vi "SP Handle Data Display Change.vi"(4 "Cache and New Are Same?":bool, 6 "Queue Cluster":T1={"Command"="", "Test Parameters"={"Stimulus"={"Use Instrument Settings"=FALSE, "Blank Frequencies"=FALSE, "Sweep Type"=enum."Linear", "Sweep"={"Fstart"=500.0, "Fstop"=1500.0, "Units"=enum."MHz", "Points"=2}, "Power (dBm)"=999.0, "IFBW (Hz)"=-1.0, "Sweep Time (s)"=-1.0, "Calibration"={"State"=FALSE, "String"=""}}, "Measurement"={"Auto Select"=TRUE, "Data Source"=enum."VNA", "Ports"=2, "Parameters"=[]}, "De-Embed"={"De-Embed"=FALSE, "Adapters"=[]}, "Display"={"Lock Control"=FALSE, "Retain Settings"=TRUE, "Formatted Data"=FALSE, "Plot Orientation"=enum."Single", "Plot Controls"=[{"Trace Orientation"=enum."Overlay", "Frequency"={"Change Frequency"=FALSE, "Start"=500.0, "Stop"=1500.0, "Units"=enum."MHz"}, "Markers"=[], "Traces"=[]}, {"Trace Orientation"=enum."Overlay", "Frequency"={"Change Frequency"=FALSE, "Start"=500.0, "Stop"=1500.0, "Units"=enum."MHz"}, "Markers"=[], "Traces"=[]}, {"Trace Orientation"=enum."Overlay", "Frequency"={"Change Frequency"=FALSE, "Start"=500.0, "Stop"=1500.0, "Units"=enum."MHz"}, "Markers"=[], "Traces"=[]}, {"Trace Orientation"=enum."Overlay", "Frequency"={"Change Frequency"=FALSE, "Start"=500.0, "Stop"=1500.0, "Units"=enum."MHz"}, "Markers"=[], "Traces"=[]}]}, "Limits"=[], "Filter Limits"=[]}} {"Test Parameters"."Filter Limits"."Parameter"."Stimulus Port" min=1 step=1; "Test Parameters"."Filter Limits"."Parameter"."Response Port" min=1 step=1; "Test Parameters"."Filter Limits"."Passband"."Bandwidth Attn" format="%.3g"; "Test Parameters"."Filter Limits"."Passband"."Stop/Span" format="%.3g"; "Test Parameters"."Filter Limits"."Passband"."Start/Center" format="%.3g"; "Test Parameters"."Measurement"."Parameters"."Channel" min=0 max=32 step=1; "Test Parameters"."Measurement"."Parameters"."Parameter"."Stimulus Port" min=1 step=1; "Test Parameters"."Measurement"."Parameters"."Parameter"."Response Port" min=1 step=1; "Test Parameters"."Limits"."Parameter"."Stimulus Port" min=1 step=1; "Test Parameters"."Limits"."Parameter"."Response Port" min=1 step=1; "Test Parameters"."Stimulus"."Sweep Time (s)" format="%.3g"; "Test Parameters"."Display"."Plot Controls"."Traces"."Reference" format="%#.2g"; "Test Parameters"."Display"."Plot Controls"."Traces"."Scale" min=0.001 step=1.0 format="%#.2g"; "Test Parameters"."Display"."Plot Controls"."Traces"."Position" min=0.0 max=10.0; "Test Parameters"."Display"."Plot Controls"."Frequency"."Stop" format="%.3g"; "Test Parameters"."Display"."Plot Controls"."Frequency"."Start" format="%.3g"}, 8 "error in (no error)":errorcluster, 9 "CH Other":refnum<vi>, 10 "CH Changing":refnum<vi>, 11 "Queue":refnum<queue>) -> (0 "error out":errorcluster, 2 "Plot?":bool)   [LabVIEW 2011]
uses:
  TypeDefs/SP Queue Cluster.ctl
  TypeDefs/SP Test Parameters.ctl
  TypeDefs/SP Stimulus Parameters.ctl
  TypeDefs/SP Frequency Units.ctl
  TypeDefs/SP Calibration State.ctl
  TypeDefs/SP Measurement.ctl
  TypeDefs/SP Parameters.ctl
  TypeDefs/SP Parameter.ctl
  TypeDefs/SP De-Embed.ctl
  TypeDefs/SP Adapter.ctl
  TypeDefs/SP Data.ctl
  TypeDefs/SP Display Parameters.ctl
  TypeDefs/SP Display Plot Controls Cluster.ctl
  TypeDefs/SP Marker Cluster.ctl
  TypeDefs/SP Marker Type.ctl
  TypeDefs/SP Display Trace Controls.ctl
  TypeDefs/SP Display Format.ctl
  TypeDefs/SP Display Data.ctl
  TypeDefs/SP Limit.ctl
  TypeDefs/SP Format.ctl
  TypeDefs/SP Limit Type.ctl
  TypeDefs/SP Limit Point.ctl
  Test Referential Limit.ctl
  TypeDefs/SP Filter.ctl
  TypeDefs/SP Filter Type.ctl
  TypeDefs/SP Filter Passband.ctl
  TypeDefs/SP Frequency Format.ctl
  TypeDefs/SP Filter Ripple.ctl
  TypeDefs/SP Attenuation Point.ctl
  TypeDefs/SP Attenuation Type.ctl
  TypeDefs/SP Skirt Rejection Point.ctl
  TypeDefs/SP Relative Loss.ctl
panel:
  # "Div"
  # "Div"
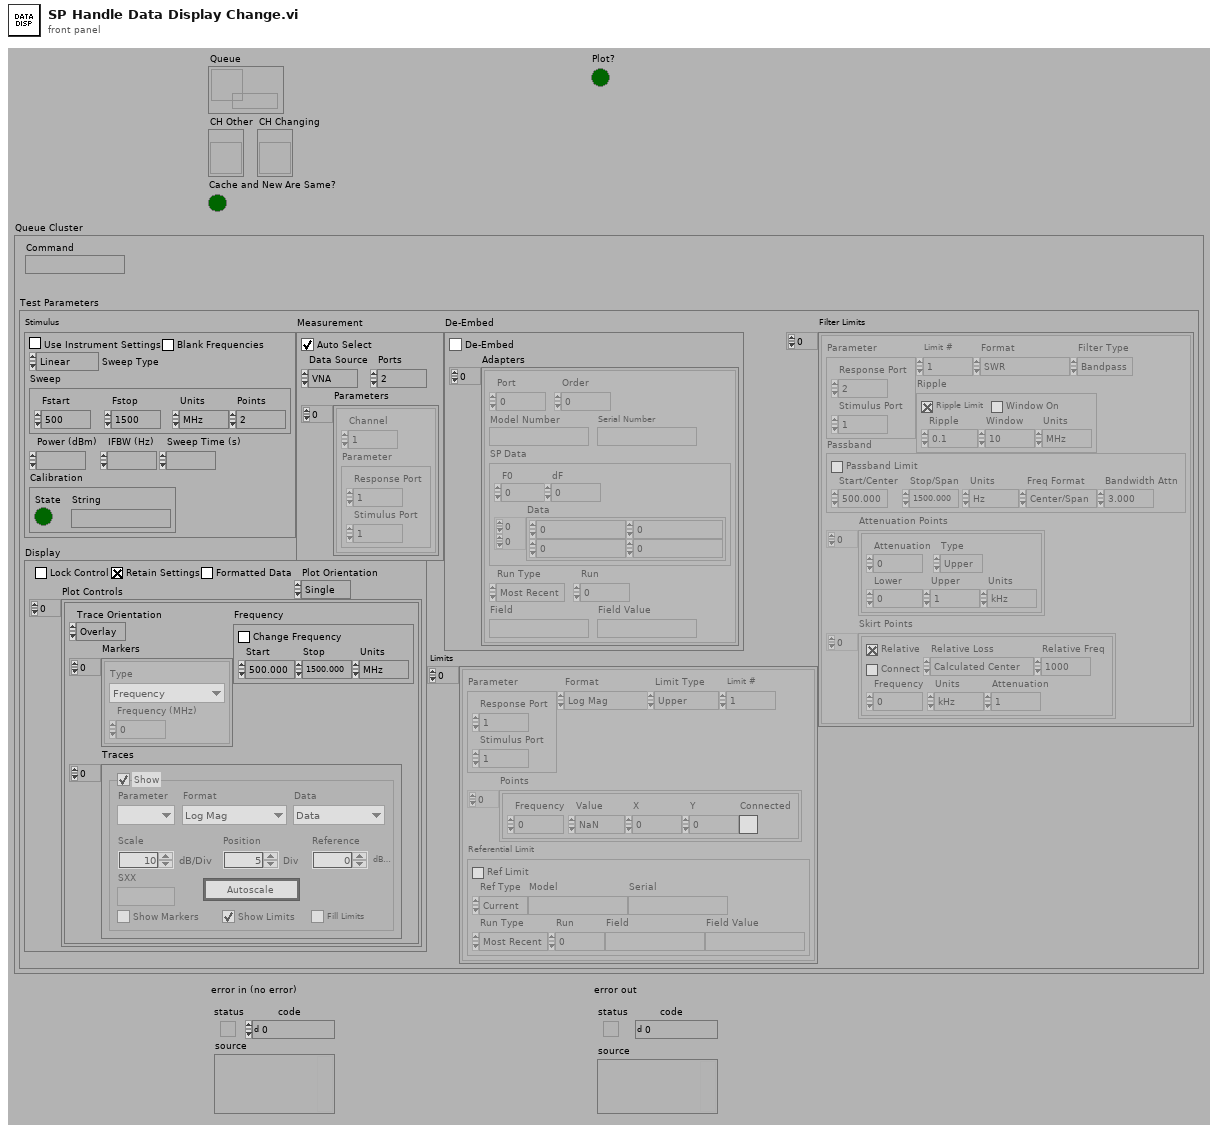
[diagram p1: front panel]
types:
  T1 = typedef "SP Queue Cluster.ctl" = cluster{"Command":string, "Test Parameters":T2}
  T2 = typedef "SP Test Parameters.ctl" = cluster{"Stimulus":T3, "Measurement":T6, "De-Embed":T9, "Display":T12, "Limits":T19[], "Filter Limits":T24[]}
  T3 = typedef "SP Stimulus Parameters.ctl" = cluster{"Use Instrument Settings":bool, "Blank Frequencies":bool, "Sweep Type":enum32{"Linear", "Logarithmic", "List", "Power", "CW"}, "Sweep":cluster{"Fstart":dbl, "Fstop":dbl, "Units":T4, "Points":i32}, "Power (dBm)":dbl, "IFBW (Hz)":dbl, "Sweep Time (s)":dbl, "Calibration":T5}
  T4 = typedef "SP Frequency Units.ctl" = enum16{"Hz", "kHz", "MHz", "GHz", "Points"}
  T5 = typedef "SP Calibration State.ctl" = cluster{"State":bool, "String":string}
  T6 = typedef "SP Measurement.ctl" = cluster{"Auto Select":bool, "Data Source":enum16{"VNA", "Data File"}, "Ports":i8, "Parameters":T7[]}
  T7 = typedef "SP Parameters.ctl" = cluster{"Channel":i8, "Parameter":T8}
  T8 = typedef "SP Parameter.ctl" = cluster{"Stimulus Port":i8, "Response Port":i8}
  T9 = typedef "SP De-Embed.ctl" = cluster{"De-Embed":bool, "Adapters":T10[]}
  T10 = typedef "SP Adapter.ctl" = cluster{"Port":i8, "Order":i8, "Model Number":string, "Serial Number":string, "SP Data":T11, "Run Type":enum16{"Most Recent", "Run #", "Match Field"}, "Run":i32, "Field":string, "Field Value":string}
  T11 = typedef "SP Data.ctl" = cluster{"F0":dbl, "dF":dbl, "Data":cdb[][]}
  T12 = typedef "SP Display Parameters.ctl" = cluster{"Lock Control":bool, "Retain Settings":bool, "Formatted Data":bool, "Plot Orientation":enum32{"Single", "Dual", "Quad"}, "Plot Controls":T13[]}
  T13 = typedef "SP Display Plot Controls Cluster.ctl" = cluster{"Trace Orientation":enum32{"Overlay", "Split"}, "Frequency":cluster{"Change Frequency":bool, "Start":dbl, "Stop":dbl, "Units":T4}, "Markers":T14[], "Traces":T16[]}
  T14 = typedef "SP Marker Cluster.ctl" = cluster{"Type":T15, "Frequency (MHz)":dbl}
  T15 = typedef "SP Marker Type.ctl" = enum16{"Frequency", "Trace Maximum", "Trace Minimum", "Limit Maximum", "Limit Minimum"}
  T16 = typedef "SP Display Trace Controls.ctl" = cluster{"Trace On":bool, "Measure":i32, "Format":T17, "Autoscale":bool, "Reference":dbl, "\nRefUnit":string, "Position":dbl, "Scale":dbl, "ScaleUnit":string, "LimitOn":bool, "LimitFill":bool, "Display Data":T18, "Show Markers":bool, "SXX":string}
  T17 = typedef "SP Display Format.ctl" = i32
  T18 = typedef "SP Display Data.ctl" = u16
  T19 = typedef "SP Limit.ctl" = cluster{"Parameter":T8, "Format":T20, "Limit Type":T21, "Points":T22[], "Referential Limit":T23, "Limit #":i8}
  T20 = typedef "SP Format.ctl" = enum16{"Log Mag", "Lin Mag", "SWR", "Phase", "Expanded Phase", "Delay", "Insertion Loss", "Isolation", "Return Loss"}
  T21 = typedef "SP Limit Type.ctl" = enum16{"Upper", "Lower", "Delta", "Filter", "Referential"}
  T22 = typedef "SP Limit Point.ctl" = cluster{"Frequency":dbl, "Value":dbl, "X":dbl, "Y":dbl, "Connected":bool}
  T23 = typedef "Test Referential Limit.ctl" = cluster{"Ref Limit":bool, "Ref Type":enum16{"Current", "Specify"}, "Model":string, "Serial":string, "Run Type":enum16{"Most Recent", "Run #", "Match Field"}, "Run":i32, "Field":string, "Field Value":string}
  T24 = typedef "SP Filter.ctl" = cluster{"Limit #":i8, "Parameter":T8, "Format":T20, "Filter Type":T25, "Passband":T26, "Ripple":T28, "Attenuation Points":T29[], "Skirt Points":T31[]}
  T25 = typedef "SP Filter Type.ctl" = enum16{"Lowpass", "Highpass", "Bandpass", "Bandstop"}
  T26 = typedef "SP Filter Passband.ctl" = cluster{"Start/Center":dbl, "Stop/Span":dbl, "Units":T4, "Freq Format":T27, "Bandwidth Attn":dbl, "Passband Limit":bool}
  T27 = typedef "SP Frequency Format.ctl" = enum16{"Start/Stop", "Center/Span"}
  T28 = typedef "SP Filter Ripple.ctl" = cluster{"Ripple Limit":bool, "Window On":bool, "Ripple":dbl, "Window":dbl, "Units":T4}
  T29 = typedef "SP Attenuation Point.ctl" = cluster{"Attenuation":dbl, "Type":T30, "Lower":dbl, "Upper":dbl, "Units":T4}
  T30 = typedef "SP Attenuation Type.ctl" = enum16{"Center", "Lower", "Upper"}
  T31 = typedef "SP Skirt Rejection Point.ctl" = cluster{"Relative":bool, "Connect":bool, "Frequency":dbl, "Units":T4, "Attenuation":dbl, "Relative Loss":T32, "Relative Freq":dbl}
  T32 = typedef "SP Relative Loss.ctl" = enum16{"Calculated Center", "Passband Minimum", "Passband Maximum", "Passband Average", "Frequency"}
  T33 = cluster{"Trace On":bool, "Measure":i32, "Format":T17, "Autoscale":bool, "Reference":dbl, "\nRefUnit":string, "Position":dbl, "Scale":dbl, "ScaleUnit":string, "LimitOn":bool, "LimitFill":bool, "Display Data":T18, "Show Markers":bool, "SXX":string}
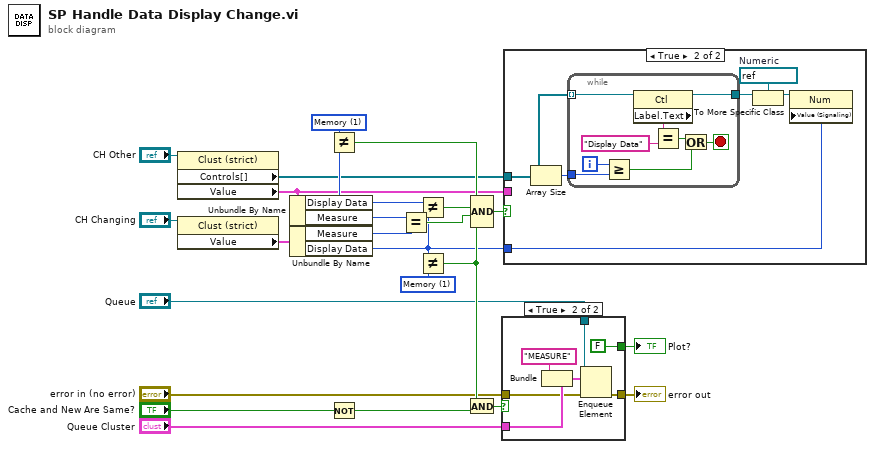
[diagram p0: block diagram]
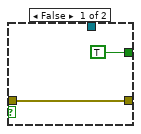
[diagram p2: hidden frame]
diagram:
  w21 = T18 1 items=["Data", "Memory", "Data/Memory"] ("y")
  w22 = T18 1 items=["Data", "Memory", "Data/Memory"] ("y")
  n1 = property class="Clust (strict)"(reference="CH Other") -> ("Controls[]"=w5:refnum<vi>[], "Value"=w13:T33)  [unwired: 1 in, 2 out]
  n2 = property class="Clust (strict)"(reference="CH Changing") -> ("Value"=w8:T33)  [unwired: 1 in, 2 out]
  n3 = Unbundle By Name(w13) -> ("Display Data"=w19:T18, "Measure"=w24:i32)
  n4 = Unbundle By Name(w8) -> ("Measure"=w23:i32, "Display Data"=w15:T18)
  n5 = Not Equal?(x=w21, y=w19) -> (x != y?=w20:bool)
  n6 = Not(x="Cache and New Are Same?") -> (.not. x?=w6:bool)
  n7 = Equal?(x=w24, y=w23) -> (x = y?=w18:bool)
  n8 = Not Equal?(x=w19, y=w15) -> (x != y?=w17:bool)
  n9 = Not Equal?(x=w15, y=w22) -> (x != y?=w16:bool)
  n10 = And(x=w16, y=w6) -> (x .and. y?=w2:bool)
  n11 = Compound Arithmetic op=AND(w20, w17, w18, w16) -> (w11:bool)
  n12 = case shown="True" w2 {
    tunnel: "Queue" -> [_ w32]
    tunnel: [w26 w31] -> w9
    tunnel: "Queue Cluster" -> [_ w30]
    tunnel: "error in (no error)" -> [w26 w29]
    tunnel: [TRUE ("Plot?") FALSE ("Plot?")] -> w1
    frame False {
    }
    frame True {
      n13 = Bundle(cluster=w30, "Command"="MEASURE") -> (w33:T1)  [unwired: 1 out]
      n14 = Enqueue Element(queue=w32, element=w33, error in (no error)=w29) -> (error out=w31:errorcluster)  [unwired: 3 out]
    }
  }
  "error out" <- w9
  "Plot?" <- w1
  n15 = case shown="True" w11 {
    tunnel: w15 -> [_ w36]
    tunnel: w13 -> [_ _]
    tunnel: w5 -> [_ w38]
    frame False {
    }
    frame True {
      w37 = refnum<vi> refnum  # Numeric
      n16 = Array Size(array=w38) -> (size(s)=w39:i32)
      n17 = while {
        tunnel: w38 -> [w48] mode=indexing
        tunnel: w39 -> [w43]
        tunnel: [w40] -> w35
        i -> [w44]
        stop <- w41 stop-if-true
        n18 = Greater Or Equal?(x=w44, y=w43) -> (x >= y?=w42:bool)
        n19 = property class="Ctl"(reference=w48) -> (reference out=w40:refnum<vi>, "Label.Text"=w47:string)  [unwired: 1 in, 1 out]
        n20 = Equal?(x=w47, y="Display Data") -> (x = y?=w45:bool)
        n21 = Or(x=w45, y=w42) -> (x .or. y?=w41:bool)
      }
      n22 = To More Specific Class(target class=w37, reference=w35) -> (specific class reference=w34:refnum<vi>)  [unwired: 1 in, 1 out]
      n23 = property class="Num"(reference=w34, "Value (Signaling)"=w36) -> ()  [unwired: 1 in, 2 out]
    }
  }
